vi "franch_toeplitz.vi"(4 "error in (no error)":errorcluster, 6 "column":cdb[](array[numeric]), 7 "row":cdb[](array[numeric])) -> (0 "error out":errorcluster, 3 "Toeplitz Array":cdb[][](array[numeric]))   [LabVIEW 2012]
uses:
  <vilib>/Analysis/7linalg.llb/Create Special Complex Matrix.vi
  <vilib>/Analysis/NI_AALPro.lvlib
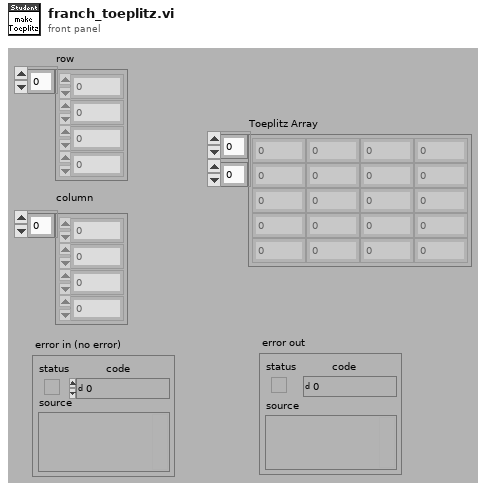
[diagram p1: front panel]
types:
  T1 = typedef "NI_Matrix.lvlib/ComplexMatrix.ctl" = cdb[][]
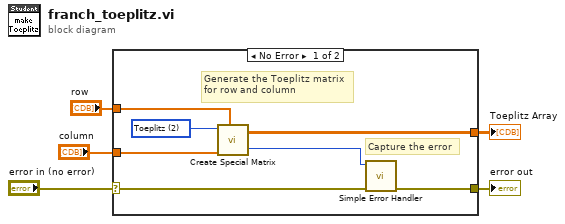
[diagram p0: block diagram]
diagram:
  n1 = case shown="No Error" "error in (no error)" {
    selector: "error in (no error)" -> [w8 w13]
    tunnel: [w11 _] -> w5
    tunnel: [w9 w13] -> w4
    tunnel: "row" -> [w7 _]
    tunnel: "column" -> [w6 _]
    frame No Error {
      w12 = 2 items=["Identity", "Diagonal", "Toeplitz", "Vandermonde", "Companion", "Hankel", "Hadamard", "Wilkinson", "Hilbert", "Inverse Hilbert", "Rosser", "Pascal"] ("matrix type")
      # "Capture the error"
      # "Generate the Toeplitz matrix\nfor row and column"
      n2 = call-poly <vilib>:"Create Special Matrix.vi"("matrix type"=w12, "Input Vector1"=w6, "Input Vector2"=w7) -> ("Special Matrix"=w11:T1, "error"=w10:i32)  [unwired: 2 in]
      n3 = call <vilib>:"Simple Error Handler.vi"("error code (no error:0)"=w10, "error in (no error)"=w8) -> ("error out"=w9:errorcluster)  [unwired: 3 in, 4 out]
    }
    frame Error {
    }
  }
  "Toeplitz Array" <- w5
  "error out" <- w4
